vi "Hardware-InitDCMRef.vi"(8 "error in (no error)":errorcluster, 9 "DCM Index (0)":i32, 11 "DCM - RT in":refnum<class "DCM - RT.lvclass">) -> (0 "error out":errorcluster, 3 "Command":T1 {"Hardware"."DCM 2"."Write"."B Profiles - Pulse Width [s]" min=0 max=0.0001 format="%#_6p"; "Hardware"."DCM 2"."Write"."A Profiles - Pulse Width [s]" min=0 max=0.0001 format="%#_6p"; "Hardware"."DCM 2"."Write"."ESTTL Setup"."Frequency [Hz]" format="%#_3p"; "Hardware"."DCM 2"."Write"."Pump B Command"."Sweep [s]" format="%#_3p"; "Hardware"."DCM 2"."Write"."Pump B Command"."Injections" max=511; "Hardware"."DCM 2"."Write"."Pump B Command"."Duration [s]" format="%#_3p"; "Hardware"."DCM 2"."Write"."Pump B Command"."Frequency [Hz]" format="%#_3p"; "Hardware"."DCM 2"."Write"."Inj B Command"."Sweep [s]" format="%#_3p"; "Hardware"."DCM 2"."Write"."Inj B Command"."Injections" max=511; "Hardware"."DCM 2"."Write"."Inj B Command"."Duration [s]" format="%#_3p"; "Hardware"."DCM 2"."Write"."Inj B Command"."Frequency [Hz]" format="%#_3p"; "Hardware"."DCM 2"."Write"."Pump A Command"."Sweep [s]" format="%#_3p"; "Hardware"."DCM 2"."Write"."Pump A Command"."Injections" max=511; "Hardware"."DCM 2"."Write"."Pump A Command"."Duration [s]" format="%#_3p"; "Hardware"."DCM 2"."Write"."Pump A Command"."Frequency [Hz]" format="%#_3p"; "Hardware"."DCM 2"."Write"."Inj A Command"."Sweep [s]" format="%#_3p"; "Hardware"."DCM 2"."Write"."Inj A Command"."Injections" max=511; "Hardware"."DCM 2"."Write"."Inj A Command"."Duration [s]" format="%#_3p"; "Hardware"."DCM 2"."Write"."Inj A Command"."Frequency [Hz]" format="%#_3p"; "Hardware"."DCM 2"."Write"."HH Cmd"."Frequency [Hz]" format="%#_3p"; "Hardware"."DCM 2"."Write"."DiffIO Setup"."Frequency [Hz]" format="%#_3p"; "Hardware"."DCM 2"."Read"."DiffIO Results"."Duty Cycle [%]" format="%#_3g"; "Hardware"."DCM 2"."Read"."DiffIO Results"."Frequency [Hz]" format="%#_3p"; "Hardware"."DCM 2"."Read"."System ADC"."12V Fan [V]" format="%#_3p"; "Hardware"."DCM 2"."Read"."System ADC"."Primary Voltage B1B2 [V]" format="%#_3p"; "Hardware"."DCM 2"."Read"."System ADC"."Primary Voltage B3B4 [V]" format="%#_3p"; "Hardware"."DCM 2"."Read"."System ADC"."Primary Voltage A3A4 [V]" format="%#_3p"; "Hardware"."DCM 2"."Read"."System ADC"."Primary Voltage A1A2 [V]" format="%#_3p"; "Hardware"."DCM 2"."Read"."System ADC"."Main Power Relay [V]" format="%#_3p"; "Hardware"."DCM 2"."Read"."System ADC"."High Voltage B [V]" format="%#_3p"; "Hardware"."DCM 2"."Read"."System ADC"."High Voltage A [V]" format="%#_3p"; "Hardware"."DCM 2"."Read"."System ADC"."Zener Aux B [V]" format="%#_3p"; "Hardware"."DCM 2"."Read"."System ADC"."Zener Aux A [V]" format="%#_3p"; "Hardware"."DCM 2"."Read"."System ADC"."Zener B [V]" format="%#_3p"; "Hardware"."DCM 2"."Read"."System ADC"."Zener A [V]" format="%#_3p"; "Hardware"."DCM 2"."Read"."System ADC"."Key [V]" format="%#_3p"; "Hardware"."DCM 2"."Read"."System ADC"."Drive Power [V]" format="%#_3p"; "Hardware"."DCM 2"."Read"."System ADC"."Battery [V]" format="%#_3p"; "Hardware"."DCM 2"."Read"."System ADC"."12V [V]" format="%#_3p"; "Hardware"."DCM 2"."Read"."System ADC"."Boost Voltage B1B2 [V]" format="%#_3p"; "Hardware"."DCM 2"."Read"."System ADC"."Boost Voltage B3B4 [V]" format="%#_3p"; "Hardware"."DCM 2"."Read"."System ADC"."Boost Voltage A3A4 [V]" format="%#_3p"; "Hardware"."DCM 2"."Read"."System ADC"."Boost Voltage A1A2 [V]" format="%#_3p"; "Hardware"."DCM 2"."Read"."System ADC"."Temp Boost B1B2 [C]" format="%#_3p"; "Hardware"."DCM 2"."Read"."System ADC"."Temp Boost B3B4 [C]" format="%#_3p"; "Hardware"."DCM 2"."Read"."System ADC"."Temp Boost A3A4 [C]" format="%#_3p"; "Hardware"."DCM 2"."Read"."System ADC"."Temp Boost A1A2 [C]" format="%#_3p"; "Hardware"."DCM 2"."Read"."System ADC"."Temp Intake [C]" format="%#_3p"; "Hardware"."DCM 2"."Read"."System ADC"."Temp CPU [C]" format="%#_3p"; "Hardware"."DCM 2"."Read"."System ADC"."Temp DI B1B2 [C]" format="%#_3p"; "Hardware"."DCM 2"."Read"."System ADC"."Temp DI B3B4 [C]" format="%#_3p"; "Hardware"."DCM 2"."Read"."System ADC"."Temp DI A3A4 [C]" format="%#_3p"; "Hardware"."DCM 2"."Read"."System ADC"."Temp DI A1A2 [C]" format="%#_3p"; "Hardware"."DCM 2"."Read"."System ADC"."Temp HH 7-12 [C]" format="%#_3p"; "Hardware"."DCM 2"."Read"."System ADC"."Temp HH 1-6 [C]" format="%#_3p"; "Hardware"."DCM 2"."Read"."System ADC"."AI 12 [V]" format="%#_3p"; "Hardware"."DCM 2"."Read"."System ADC"."AI 11 [V]" format="%#_3p"; "Hardware"."DCM 2"."Read"."System ADC"."AI 10 [V]" format="%#_3p"; "Hardware"."DCM 2"."Read"."System ADC"."AI 9 [V]" format="%#_3p"; "Hardware"."DCM 2"."Read"."System ADC"."AI 8 [V]" format="%#_3p"; "Hardware"."DCM 2"."Read"."System ADC"."AI 7 [V]" format="%#_3p"; "Hardware"."DCM 2"."Read"."System ADC"."AI 6 [V]" format="%#_3p"; "Hardware"."DCM 2"."Read"."System ADC"."AI 5 [V]" format="%#_3p"; "Hardware"."DCM 2"."Read"."System ADC"."AI 4 [V]" format="%#_3p"; "Hardware"."DCM 2"."Read"."System ADC"."AI 3 [V]" format="%#_3p"; "Hardware"."DCM 2"."Read"."System ADC"."AI 2 [V]" format="%#_3p"; "Hardware"."DCM 2"."Read"."System ADC"."AI 1 [V]" format="%#_3p"; "Hardware"."DCM 1"."Write"."B Profiles - Pulse Width [s]" min=0 max=0.0001 format="%#_6p"; "Hardware"."DCM 1"."Write"."A Profiles - Pulse Width [s]" min=0 max=0.0001 format="%#_6p"; "Hardware"."DCM 1"."Write"."ESTTL Setup"."Frequency [Hz]" format="%#_3p"; "Hardware"."DCM 1"."Write"."Pump B Command"."Sweep [s]" format="%#_3p"; "Hardware"."DCM 1"."Write"."Pump B Command"."Injections" max=511; "Hardware"."DCM 1"."Write"."Pump B Command"."Duration [s]" format="%#_3p"; "Hardware"."DCM 1"."Write"."Pump B Command"."Frequency [Hz]" format="%#_3p"; "Hardware"."DCM 1"."Write"."Inj B Command"."Sweep [s]" format="%#_3p"; "Hardware"."DCM 1"."Write"."Inj B Command"."Injections" max=511; "Hardware"."DCM 1"."Write"."Inj B Command"."Duration [s]" format="%#_3p"; "Hardware"."DCM 1"."Write"."Inj B Command"."Frequency [Hz]" format="%#_3p"; "Hardware"."DCM 1"."Write"."Pump A Command"."Sweep [s]" format="%#_3p"; "Hardware"."DCM 1"."Write"."Pump A Command"."Injections" max=511; "Hardware"."DCM 1"."Write"."Pump A Command"."Duration [s]" format="%#_3p"; "Hardware"."DCM 1"."Write"."Pump A Command"."Frequency [Hz]" format="%#_3p"; "Hardware"."DCM 1"."Write"."Inj A Command"."Sweep [s]" format="%#_3p"; "Hardware"."DCM 1"."Write"."Inj A Command"."Injections" max=511; "Hardware"."DCM 1"."Write"."Inj A Command"."Duration [s]" format="%#_3p"; "Hardware"."DCM 1"."Write"."Inj A Command"."Frequency [Hz]" format="%#_3p"; "Hardware"."DCM 1"."Write"."HH Cmd"."Frequency [Hz]" format="%#_3p"; "Hardware"."DCM 1"."Write"."DiffIO Setup"."Frequency [Hz]" format="%#_3p"; "Hardware"."DCM 1"."Read"."DiffIO Results"."Duty Cycle [%]" format="%#_3g"; "Hardware"."DCM 1"."Read"."DiffIO Results"."Frequency [Hz]" format="%#_3p"; "Hardware"."DCM 1"."Read"."System ADC"."12V Fan [V]" format="%#_3p"; "Hardware"."DCM 1"."Read"."System ADC"."Primary Voltage B1B2 [V]" format="%#_3p"; "Hardware"."DCM 1"."Read"."System ADC"."Primary Voltage B3B4 [V]" format="%#_3p"; "Hardware"."DCM 1"."Read"."System ADC"."Primary Voltage A3A4 [V]" format="%#_3p"; "Hardware"."DCM 1"."Read"."System ADC"."Primary Voltage A1A2 [V]" format="%#_3p"; "Hardware"."DCM 1"."Read"."System ADC"."Main Power Relay [V]" format="%#_3p"; "Hardware"."DCM 1"."Read"."System ADC"."High Voltage B [V]" format="%#_3p"; "Hardware"."DCM 1"."Read"."System ADC"."High Voltage A [V]" format="%#_3p"; "Hardware"."DCM 1"."Read"."System ADC"."Zener Aux B [V]" format="%#_3p"; "Hardware"."DCM 1"."Read"."System ADC"."Zener Aux A [V]" format="%#_3p"; "Hardware"."DCM 1"."Read"."System ADC"."Zener B [V]" format="%#_3p"; "Hardware"."DCM 1"."Read"."System ADC"."Zener A [V]" format="%#_3p"; "Hardware"."DCM 1"."Read"."System ADC"."Key [V]" format="%#_3p"; "Hardware"."DCM 1"."Read"."System ADC"."Drive Power [V]" format="%#_3p"; "Hardware"."DCM 1"."Read"."System ADC"."Battery [V]" format="%#_3p"; "Hardware"."DCM 1"."Read"."System ADC"."12V [V]" format="%#_3p"; "Hardware"."DCM 1"."Read"."System ADC"."Boost Voltage B1B2 [V]" format="%#_3p"; "Hardware"."DCM 1"."Read"."System ADC"."Boost Voltage B3B4 [V]" format="%#_3p"; "Hardware"."DCM 1"."Read"."System ADC"."Boost Voltage A3A4 [V]" format="%#_3p"; "Hardware"."DCM 1"."Read"."System ADC"."Boost Voltage A1A2 [V]" format="%#_3p"; "Hardware"."DCM 1"."Read"."System ADC"."Temp Boost B1B2 [C]" format="%#_3p"; "Hardware"."DCM 1"."Read"."System ADC"."Temp Boost B3B4 [C]" format="%#_3p"; "Hardware"."DCM 1"."Read"."System ADC"."Temp Boost A3A4 [C]" format="%#_3p"; "Hardware"."DCM 1"."Read"."System ADC"."Temp Boost A1A2 [C]" format="%#_3p"; "Hardware"."DCM 1"."Read"."System ADC"."Temp Intake [C]" format="%#_3p"; "Hardware"."DCM 1"."Read"."System ADC"."Temp CPU [C]" format="%#_3p"; "Hardware"."DCM 1"."Read"."System ADC"."Temp DI B1B2 [C]" format="%#_3p"; "Hardware"."DCM 1"."Read"."System ADC"."Temp DI B3B4 [C]" format="%#_3p"; "Hardware"."DCM 1"."Read"."System ADC"."Temp DI A3A4 [C]" format="%#_3p"; "Hardware"."DCM 1"."Read"."System ADC"."Temp DI A1A2 [C]" format="%#_3p"; "Hardware"."DCM 1"."Read"."System ADC"."Temp HH 7-12 [C]" format="%#_3p"; "Hardware"."DCM 1"."Read"."System ADC"."Temp HH 1-6 [C]" format="%#_3p"; "Hardware"."DCM 1"."Read"."System ADC"."AI 12 [V]" format="%#_3p"; "Hardware"."DCM 1"."Read"."System ADC"."AI 11 [V]" format="%#_3p"; "Hardware"."DCM 1"."Read"."System ADC"."AI 10 [V]" format="%#_3p"; "Hardware"."DCM 1"."Read"."System ADC"."AI 9 [V]" format="%#_3p"; "Hardware"."DCM 1"."Read"."System ADC"."AI 8 [V]" format="%#_3p"; "Hardware"."DCM 1"."Read"."System ADC"."AI 7 [V]" format="%#_3p"; "Hardware"."DCM 1"."Read"."System ADC"."AI 6 [V]" format="%#_3p"; "Hardware"."DCM 1"."Read"."System ADC"."AI 5 [V]" format="%#_3p"; "Hardware"."DCM 1"."Read"."System ADC"."AI 4 [V]" format="%#_3p"; "Hardware"."DCM 1"."Read"."System ADC"."AI 3 [V]" format="%#_3p"; "Hardware"."DCM 1"."Read"."System ADC"."AI 2 [V]" format="%#_3p"; "Hardware"."DCM 1"."Read"."System ADC"."AI 1 [V]" format="%#_3p"})   [LabVIEW 2015]
uses:
  <vilib>/Powertrain Controls/Device Drivers/DCM/Rev0/RT/DCM - RT.lvclass
  Typedefs/Command.ctl
  Typedefs/Command-Hardware.ctl
  Typedefs/Command-Hardware-DCM.ctl
  Typedefs/Command-Hardware-DCM-Read.ctl
  <vilib>/Powertrain Controls/Device Drivers/DCM/Rev0/RT/System ADC.ctl
  <vilib>/Powertrain Controls/Device Drivers/DCM/Diff IO/RT/Results.ctl
  <vilib>/Powertrain Controls/Device Drivers/Engine Position Tracking/EPTx/RevA/RT/Controls/EPTxData.ctl
  Typedefs/Command-Hardware-DCM-Write.ctl
  <vilib>/Powertrain Controls/Device Drivers/DCM/Diff IO/RT/Setup.ctl
  <vilib>/Powertrain Controls/Device Drivers/DCM/Diff IO/FPGA/Mode.ctl
  <vilib>/Powertrain Controls/Device Drivers/DCM/Diff IO/RT/Angle Control.ctl
  <vilib>/Powertrain Controls/Device Drivers/DCM/HH/RT/Config.ctl
  <vilib>/Powertrain Controls/Device Drivers/DCM/HH/RT/Mode.ctl
  <vilib>/Powertrain Controls/Device Drivers/DCM/HH/RT/ISeq.ctl
  <vilib>/Powertrain Controls/Device Drivers/DCM/HH/RT/Setup.ctl
  <vilib>/Powertrain Controls/Device Drivers/DCM/HH/FPGA/Mode.ctl
  <vilib>/Powertrain Controls/Device Drivers/DCM/Rev0/FPGA/Digital Channel.ctl
  <vilib>/Powertrain Controls/Device Drivers/DCM/HH/RT/Angle Control.ctl
  <vilib>/Powertrain Controls/Device Drivers/DCM/DI/RT/Command.ctl
  <vilib>/Powertrain Controls/Device Drivers/DCM/DI/FPGA/Mode.ctl
  <vilib>/Powertrain Controls/Device Drivers/DCM/DI/RT/Command Sequence.ctl
  <vilib>/Powertrain Controls/Device Drivers/DCM/DI/RT/Angle Control.ctl
  <vilib>/Powertrain Controls/Device Drivers/DCM/ESTTL/RT/Setup.ctl
  <vilib>/Powertrain Controls/Device Drivers/DCM/ESTTL/FPGA/Mode.ctl
  <vilib>/Powertrain Controls/Device Drivers/DCM/ESTTL/RT/Angle Control.ctl
  Typedefs/Engine.ctl
  Typedefs/Engine-AIChannel.ctl
  Typedefs/Control.ctl
  Typedefs/Engine-RPC-Control.ctl
  Typedefs/Control-DIFuel-Control.ctl
  DSI-RT.lvlib
  <vilib>/Powertrain Controls/Device Drivers/DCM/ESTTL/RT/DCM - RT - ESTTL.lvlib
  <vilib>/Powertrain Controls/Device Drivers/DCM/ESTTL/FPGA/DCM - FPGA - ESTTL.lvlib
  <vilib>/Powertrain Controls/Device Drivers/DCM/DI/RT/DCM - RT - DI.lvlib
  <vilib>/Powertrain Controls/Device Drivers/DCM/Rev0/FPGA/DCM - FPGA.lvlib
  <vilib>/Powertrain Controls/Device Drivers/DCM/DI/FPGA/DCM - FPGA - DI.lvlib
  <vilib>/Powertrain Controls/Device Drivers/DCM/HH/RT/DCM - RT - HH.lvlib
  <vilib>/Powertrain Controls/Device Drivers/DCM/HH/FPGA/DCM - FPGA - HH.lvlib
  <vilib>/Powertrain Controls/Device Drivers/DCM/Diff IO/RT/DCM - RT - Diff IO.lvlib
  <vilib>/Powertrain Controls/Device Drivers/DCM/Diff IO/FPGA/DCM - FPGA - Diff IO.lvlib
  <vilib>/Powertrain Controls/Device Drivers/Engine Position Tracking/EPTx/RevA/RT/EPTx - RevA - RT.lvlib
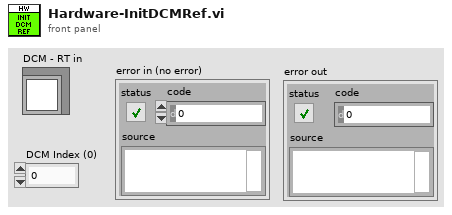
[diagram p1: front panel]
types:
  T1 = typedef "DSI-RT.lvlib/Command.ctl" = cluster{"dt(s)":sgl, "Hardware":T2, "Engine":T26, "Control":T28}
  T2 = typedef "DSI-RT.lvlib/Command-Hardware.ctl" = cluster{"DCM 1":T3, "DCM 2":T3}
  T3 = typedef "DSI-RT.lvlib/Command-Hardware-DCM.ctl" = cluster{"DCM Ref":refnum<class "DCM - RT.lvclass">, "Read":T4, "Write":T8}
  T4 = typedef "DSI-RT.lvlib/Command-Hardware-DCM-Read.ctl" = cluster{"System ADC":T5, "DiffIO Results":T6[], "EPTxData":T7, "Knock Results":cluster{"Knock":bool[], "Knock Intensity":sgl[]}, "DiffIO State":bool[]}
  T5 = typedef "DCM - RT.lvclass/System ADC.ctl" = cluster{"AI 1 [V]":sgl, "AI 2 [V]":sgl, "AI 3 [V]":sgl, "AI 4 [V]":sgl, "AI 5 [V]":sgl, "AI 6 [V]":sgl, "AI 7 [V]":sgl, "AI 8 [V]":sgl, "AI 9 [V]":sgl, "AI 10 [V]":sgl, "AI 11 [V]":sgl, "AI 12 [V]":sgl, "Temp HH 1-6 [C]":sgl, "Temp HH 7-12 [C]":sgl, "Temp DI A1A2 [C]":sgl, "Temp DI A3A4 [C]":sgl, "Temp DI B3B4 [C]":sgl, "Temp DI B1B2 [C]":sgl, "Temp CPU [C]":sgl, "Temp Intake [C]":sgl, "Temp Boost A1A2 [C]":sgl, "Temp Boost A3A4 [C]":sgl, "Temp Boost B3B4 [C]":sgl, "Temp Boost B1B2 [C]":sgl, "Primary Voltage A1A2 [V]":sgl, "Primary Voltage A3A4 [V]":sgl, "Primary Voltage B3B4 [V]":sgl, "Primary Voltage B1B2 [V]":sgl, "Boost Voltage A1A2 [V]":sgl, "Boost Voltage A3A4 [V]":sgl, "Boost Voltage B3B4 [V]":sgl, "Boost Voltage B1B2 [V]":sgl, "High Voltage A [V]":sgl, "High Voltage B [V]":sgl, "12V [V]":sgl, "12V Fan [V]":sgl, "Battery [V]":sgl, "Drive Power [V]":sgl, "Key [V]":sgl, "Zener A [V]":sgl, "Zener B [V]":sgl, "Zener Aux A [V]":sgl, "Zener Aux B [V]":sgl, "Main Power Relay [V]":sgl}
  T6 = typedef "DCM - RT - Diff IO.lvlib/Results.ctl" = cluster{"Capture [DBTDC]":sgl, "Capture Error":bool, "Frequency [Hz]":sgl, "Duty Cycle [%]":sgl, "PWM Stopped":bool}
  T7 = typedef "EPTx - RevA - RT.lvlib/EPTxData.ctl" = cluster{"Sync":bool, "CurrentCAD":sgl, "Speed [RPM]":sgl, "Config":bool, "Rcvg Primary":bool, "Stall":bool, "Overflow":bool, "Ratio Error":bool, "Pattern Error":bool, "Aux Warning":bool, "Watchdog Error":bool}
  T8 = typedef "DSI-RT.lvlib/Command-Hardware-DCM-Write.ctl" = cluster{"DiffIO Setup":T9[], "HH Config":T12[], "HH Cmd":T15[], "Inj A Command":T19[], "Pump A Command":T19, "Inj B Command":T19[], "Pump B Command":T19, "UEGO1 Disable":bool, "UEGO2 Disable":bool, "ESTTL Setup":T23[], "A Profiles - Pulse Width [s]":sgl[][], "B Profiles - Pulse Width [s]":sgl[][]}
  T9 = typedef "DCM - RT - Diff IO.lvlib/Setup.ctl" = cluster{"Mode":T10, "Capture Start [DBTDC]":sgl, "Capture End [DBTDC]":sgl, "Polarity":bool, "Frequency [Hz]":sgl, "Duty Cycle [%]":sgl, "TDC Offset [CAD]":sgl, "Window Start [DBTDC]":sgl, "Window End [DBTDC]":sgl, "Angles":T11[], "Skip Fire":bool, "Total Cycles":u8, "On Cycles":u8}
  T10 = typedef "DCM - FPGA - Diff IO.lvlib/Mode.ctl" = enum8{"Off", "Input", "Pulse Width Modulation", "Engine Position Tracking"}
  T11 = typedef "DCM - RT - Diff IO.lvlib/Angle Control.ctl" = cluster{"Enable":bool, "Location [DBTDC]":sgl, "Duration [s]":sgl}
  T12 = typedef "DCM - RT - HH.lvlib/Config.ctl" = cluster{"Mode":T13, "IO Lock State":bool, "Phase 1 FP":bool, "Fault Clear":bool, "ISeq":T14[]}
  T13 = typedef "DCM - RT - HH.lvlib/Mode.ctl" = enum16{"Off", "Lowside", "Highside", "PFI", "Full H", "3-Phase"}
  T14 = typedef "DCM - RT - HH.lvlib/ISeq.ctl" = cluster{"Upper [A]":sgl, "Lower [A]":sgl, "Duration [s]":sgl}
  T15 = typedef "DCM - RT - HH.lvlib/Setup.ctl" = cluster{"Mode":T16, "Digital Input":T17, "Polarity":bool, "Frequency [Hz]":sgl, "Duty Cycle [%]":sgl, "TDC Offset [CAD]":sgl, "Window Start [DBTDC]":sgl, "Window End [DBTDC]":sgl, "Angles":T18[], "Skip Fire":bool, "Total Cycles":u8, "On Cycles":u8}
  T16 = typedef "DCM - FPGA - HH.lvlib/Mode.ctl" = enum8{"Off", "Direct", "Pulse Width Modulation", "Engine Position Tracking"}
  T17 = typedef "DCM - FPGA.lvlib/Digital Channel.ctl" = enum8{"Unused", "Diff IO 1", "Diff IO 2", "Diff IO 3", "Diff IO 4", "Diff IO 5", "Diff IO 6", "Diff IO 7", "Diff IO 8", "Aux 1", "Aux 2", "Aux 3", "Aux 4", "Aux 5", "Aux 6", "Aux 7", "Aux 8", "User OS"}
  T18 = typedef "DCM - RT - HH.lvlib/Angle Control.ctl" = cluster{"Enable":bool, "Location [DBTDC]":sgl, "Duration [s]":sgl}
  T19 = typedef "DCM - RT - DI.lvlib/Command.ctl" = cluster{"Mode":T20, "Digital Input":T17, "Frequency [Hz]":sgl, "Duration [s]":sgl, "Sweep [s]":sgl, "Injections":u16, "Command Sequence":T21[], "TDC Offset [CAD]":sgl, "Window Start [DBTDC]":sgl, "Window End [DBTDC]":sgl, "Angles":T22[], "Skip Fire":bool, "Total Cycles":u8, "On Cycles":u8}
  T20 = typedef "DCM - FPGA - DI.lvlib/Mode.ctl" = enum8{"Off", "Direct", "Calibration", "Triggered Multi-Pulse", "Engine Position Tracking"}
  T21 = typedef "DCM - RT - DI.lvlib/Command Sequence.ctl" = cluster{"Duration [s]":sgl, "CmdLevel":bool, "Continue":bool, "Phase Index":u8}
  T22 = typedef "DCM - RT - DI.lvlib/Angle Control.ctl" = cluster{"Enable":bool, "Location [DBTDC]":sgl, "Duration [s]":sgl, "Phase Index":u8}
  T23 = typedef "DCM - RT - ESTTL.lvlib/Setup.ctl" = cluster{"Mode":T24, "Polarity":bool, "Frequency [Hz]":sgl, "Duty Cycle [%]":sgl, "TDC Offset [CAD]":sgl, "Window Start [DBTDC]":sgl, "Window End [DBTDC]":sgl, "Angles":T25[], "Skip Fire":bool, "Total Cycles":u8, "On Cycles":u8}
  T24 = typedef "DCM - FPGA - ESTTL.lvlib/Mode.ctl" = enum8{"Off", "Pulse Width Modulation", "Engine Position Tracking"}
  T25 = typedef "DCM - RT - ESTTL.lvlib/Angle Control.ctl" = cluster{"Enable":bool, "Location [DBTDC]":sgl, "Duration [s]":sgl}
  T26 = typedef "DSI-RT.lvlib/Engine.ctl" = cluster{"Sensors":T27[]}
  T27 = typedef "DSI-RT.lvlib/Engine-AIChannel.ctl" = cluster{"Name":string, "Unit":string, "Value":sgl}
  T28 = typedef "DSI-RT.lvlib/Control.ctl" = cluster{"RPC":T29, "DI":T30}
  T29 = typedef "DSI-RT.lvlib/Engine-RPC-Control.ctl" = cluster{"RailP SetPoint [bar]":sgl, "RailP [bar]":sgl[], "Cam Position [CAD]":sgl[], "High Pressure Fault":bool, "TotalFuelQty [mm3/cycle]":sgl, "Pump Trig Period [sec]":sgl[], "PumpDigInputSelect":T17[]}
  T30 = typedef "DSI-RT.lvlib/Control-DIFuel-Control.ctl" = cluster{"InjectionQtys\n[mm3/stroke]":sgl[][]}
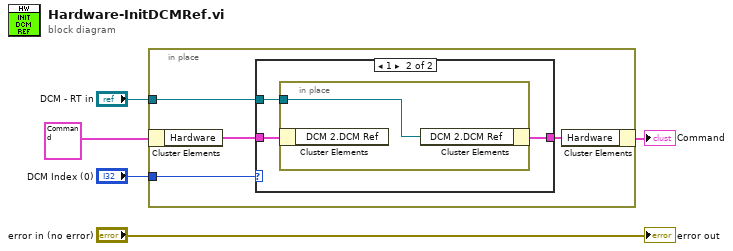
[diagram p0: block diagram]
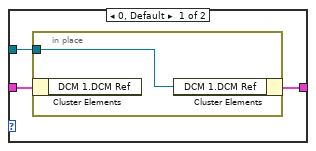
[diagram p2: hidden frame]
diagram:
  n1 = in-place {
    in-place-border: "DCM - RT in" -> [w9]
    in-place-border: "DCM Index (0)" -> [w6]
    n2 = in-place-cluster #1(T1 data[31815B] ("Command")) -> ("Hardware"=w8:T2)
    n3 = case shown="1" w6 {
      tunnel: w9 -> [w12 w16]
      tunnel: w8 -> [w11 w15]
      tunnel: [w10 w14] -> w7
      frame 0, Default {
        n4 = in-place {
          in-place-border: w12 -> [w13]
          n5 = in-place-cluster #2(w11) -> ()  [unwired: 1 out]
          n6 = in-place-cluster #2("DCM 1.DCM Ref"=w13) -> (w10:T2)
        }
      }
      frame 1 {
        n7 = in-place {
          in-place-border: w16 -> [w17]
          n8 = in-place-cluster #3(w15) -> ()  [unwired: 1 out]
          n9 = in-place-cluster #3("DCM 2.DCM Ref"=w17) -> (w14:T2)
        }
      }
    }
    n10 = in-place-cluster #1("Hardware"=w7) -> (→"Command":T1)
  }
  "error out" <- "error in (no error)"
